vi "TeleopTest.vi"(11 "Call Context":T5) -> ()   [LabVIEW 2015]
doc: "This VI is called for each TeleOp packet received from the DS where the robot is not disabled. It is often used to read from the joysticks and update I/O or to update setpoints for timed control loops. It should complete and return within 20 milliseconds or it may miss DS packets."
uses:
  <vilib>/Rock Robotics/WPI/DriverStation/WPI_DriverStationDerivedRobotMode.ctl
  <vilib>/Rock Robotics/WPI/CAN/TalonSRX/WPI_CANTalonSRX_APIControlMode.ctl
  <vilib>/Rock Robotics/WPI/Utilities/WPI_GetSetVariantRefNum.vi
  Robot Global Data.vi
panel:
  out "error out":errorcluster
  in  "Tab Control":T1(tab)
  out "Maximum":dbl
  out "Minimum":dbl
  out "Maximum?":bool
  out "Minimum?":bool
  in  "Max Length":dbl
  out "Length/Data":dbl
  in  "Angle":dbl(knob) scale=0.0..60.0
  in  "LA PID":cluster{"P":dbl, "I":dbl, "D":dbl}
  in  "Other Settings":T2
  in  "Frequency":dbl
  out "ZN PID":cluster{"P":dbl, "I":dbl, "D":dbl}
  in  "Other Settings":T2
  in  "Wheel PID":cluster{"P":dbl, "I":dbl, "D":dbl}
  in  "Ticks/100ms":dbl
  in  "Frequency":dbl
  out "ZN PID":cluster{"P":dbl, "I":dbl, "D":dbl}
  out "Trigger":bool
  out "Collection Trigger":bool
  out "Lower Button":bool
  out "Vision Prep Button":bool
  out "Motor Position":dbl
  out "Launch Speed":dbl
  in  "Cluster":T3={"LA Distance/Tick(inches)"=0.0, "Framerate"=1000, "Initial Velocity"=0.0, "Max Angle"=60, "Sims/angle"=10}
  in  "Aimbot Transformations":T4={"SpinupDuration(10ms)"=100, "ShotDuration(10ms)"=100, "PowerScale"=1.0, "AngleShift"=0}
  out "Vision Prep Button":bool
  out "Lower Button":bool
  in  "Distance":dbl
  out "Vision Distance":dbl
  out "Launch Speed":dbl
  out "Motor Position":dbl
  out "Trigger":bool
  out "Collection Trigger":bool
  in  "Aimbot Transformations":T4={"SpinupDuration(10ms)"=100, "ShotDuration(10ms)"=100, "PowerScale"=1.0, "AngleShift"=0}
  out "Collection Trigger":bool
  out "Trigger":bool
  out "Lower Button":bool
  out "Vision Prep Button":bool
  out "Launch Speed":dbl
  out "Motor Position":dbl
  out "Vision Distance":dbl
  in  "error in (no error)":errorcluster
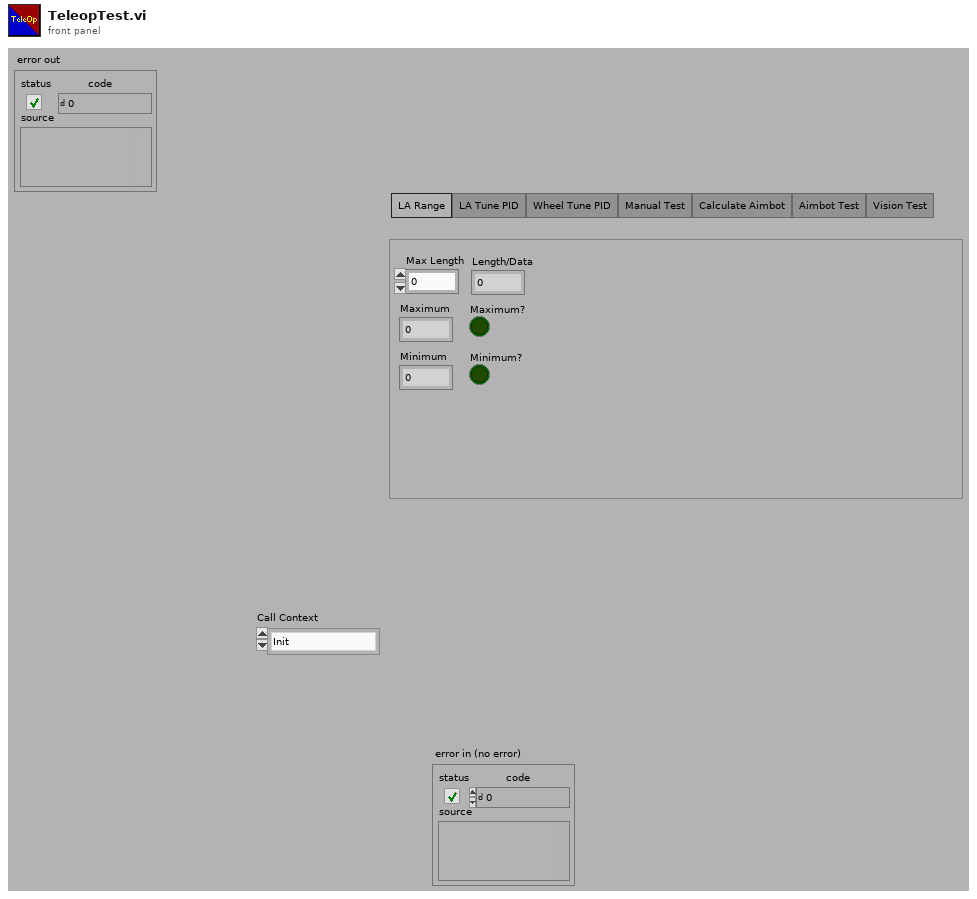
[diagram p1: front panel]
types:
  T1 = enum32{"LA Range", "LA Tune PID", "Wheel Tune PID", "Manual Test", "Calculate Aimbot", "Aimbot Test", "Vision Test"}
  T2 = cluster{"Parameter Slot":u8, "F":dbl, "I Zone":dbl, "Ramp Rate":dbl}
  T3 = cluster{"LA Distance/Tick(inches)":dbl, "Framerate":i32, "Initial Velocity":dbl, "Max Angle":i32, "Sims/angle":i32}
  T4 = cluster{"SpinupDuration(10ms)":i32, "ShotDuration(10ms)":i32, "PowerScale":dbl, "AngleShift":i32}
  T5 = typedef "WPI_DriverStationDerivedRobotMode.ctl" = enum16{"Init", "Execute", "Stop"}
  T6 = typedef "WPI_JoystickDevRef.ctl" = cluster{"Device":T7}
  T7 = typedef "WPI_JoystickDeviceEnum.ctl" = enum16{"USB 0", "USB 1", "USB 2", "USB 3", "USB 4", "USB 5"}
  T8 = typedef "WPI_CANTalonSRX_APIControlMode.ctl" = enum8{"Percent VBus", "Speed", "Position", "Slave", "Unchanged / Invalid", "Voltage Compensation", "Current", "Motion Profile"}
  T9 = cluster{"Joystick":dbl, "LowerButton":bool, "VisionPrepButton":bool, "Aimbot?":bool}
  T10 = cluster{"Framerate":i32, "Initial Velocity":dbl, "Max Angle":i32, "Min Angle":i32, "Sims/angle":i32, "Full Path":path, "Partial Path":path}
  T11 = cluster{"Ball Diameter(in)":dbl, "Air Density(g/in^3)":dbl, "Drag coefficient":dbl, "Ball Mass(g)":dbl, "gravity(in/s^2)":dbl, "Minimum Goal Height(in)":dbl, "Maximum Goal Height(in)":dbl}
  T12 = cluster{"Distance from Pivot Point to Drive Mount(in)":dbl, "Distance from Pivot Point to Arm Mount(in)":dbl, "Distance from Pivot Point to Launcher(in)":dbl, "Distance from Pivot Point to Camera(in)":dbl, "WheelEncoder Ticks/Revolution":dbl, "Wheel Radius":dbl, "Triangle Angle(degrees)":dbl, "Minimum LA Distance(inches)":dbl, "LA Distance/Tick(inches)":dbl}
  T13 = cluster{"Axes[0]":dbl, "Axes[1]":dbl, "Axes[2]":dbl, "Axes[3]":dbl, "Axes[4]":dbl, "Axes[5]":dbl, "Axes[6]":dbl, "Axes[7]":dbl, "Axes[8]":dbl}
  T14 = typedef "WPI_DigitalInputDevRef.ctl" = cluster{"DevStatus":errorcluster, "DIO Channel":T15}
  T15 = typedef "FPGA_DIOChannel.ctl" = enum8{"DIO 0", "DIO 1", "DIO 2", "DIO 3", "DIO 4", "DIO 5", "DIO 6", "DIO 7", "DIO 8", "DIO 9", "DIO MXP 0", "DIO MXP 1", "DIO MXP 2", "DIO MXP 3", "DIO MXP 4", "DIO MXP 5", "DIO MXP 6", "DIO MXP 7", "DIO MXP 8", "DIO MXP 9", "DIO MXP 10", "DIO MXP 11", "DIO MXP 12", "DIO MXP 13", "DIO MXP 14", "DIO MXP 15", "Invalid"}
  T16 = typedef "WPI_MotorControlDeviceRef.ctl" = cluster{"DeviceStatus":errorcluster, "Type":T17, "PWM":cluster{"PWM Channel":T18, "DeadBand":T19}, "CAN":cluster{"Device Number":u8, "Control Mode":T20, "Semaphore":T21, "Max Vout":dbl, "TalonSRX Control Mode":T8}, "Invert":bool}
  T17 = typedef "WPI_MotorControlType.ctl" = enum16{"PWM", "CAN", "CANTalonSRX"}
  T18 = typedef "FPGA_DIOPWMChannel.ctl" = enum8{"PWM 0", "PWM 1", "PWM 2", "PWM 3", "PWM 4", "PWM 5", "PWM 6", "PWM 7", "PWM 8", "PWM 9", "PWM MXP 0", "PWM MXP 1", "PWM MXP 2", "PWM MXP 3", "PWM MXP 4", "PWM MXP 5", "PWM MXP 6", "PWM MXP 7", "PWM MXP 8", "PWM MXP 9", "Invalid"}
  T19 = typedef "WPI_PWMDeadband.ctl" = cluster{"Name":string, "maxPositivePwm":i32, "minPositivePwm":i32, "centerPwm":i32, "maxNegativePwm":i32, "minNegativePwm":i32, "angularRange":u16}
  T20 = typedef "WPI_CANJaguar_ControlMode.ctl" = enum8{"Percent VBus", "Current", "Speed", "Position", "Voltage"}
  T21 = typedef "Semaphore RefNum" = refnum<k1>
  T22 = typedef "WPI_PotentiometerDevRef.ctl" = cluster{"DevStatus":errorcluster, "Analog Channel":T23, "Invert Output":bool}
  T23 = typedef "FPGA_AIChannel.ctl" = enum8{"AI 0", "AI 1", "AI 2", "AI 3", "AI MXP 0", "AI MXP 1", "AI MXP 2", "AI MXP 3", "Invalid"}
  T24 = cluster{"Buttons[0]":bool, "Buttons[1]":bool, "Buttons[2]":bool, "Buttons[3]":bool, "Buttons[4]":bool, "Buttons[5]":bool, "Buttons[6]":bool, "Buttons[7]":bool, "Buttons[8]":bool}
  T25 = cluster{"Angle":dbl, "Distance":dbl, "x":dbl, "y":dbl}
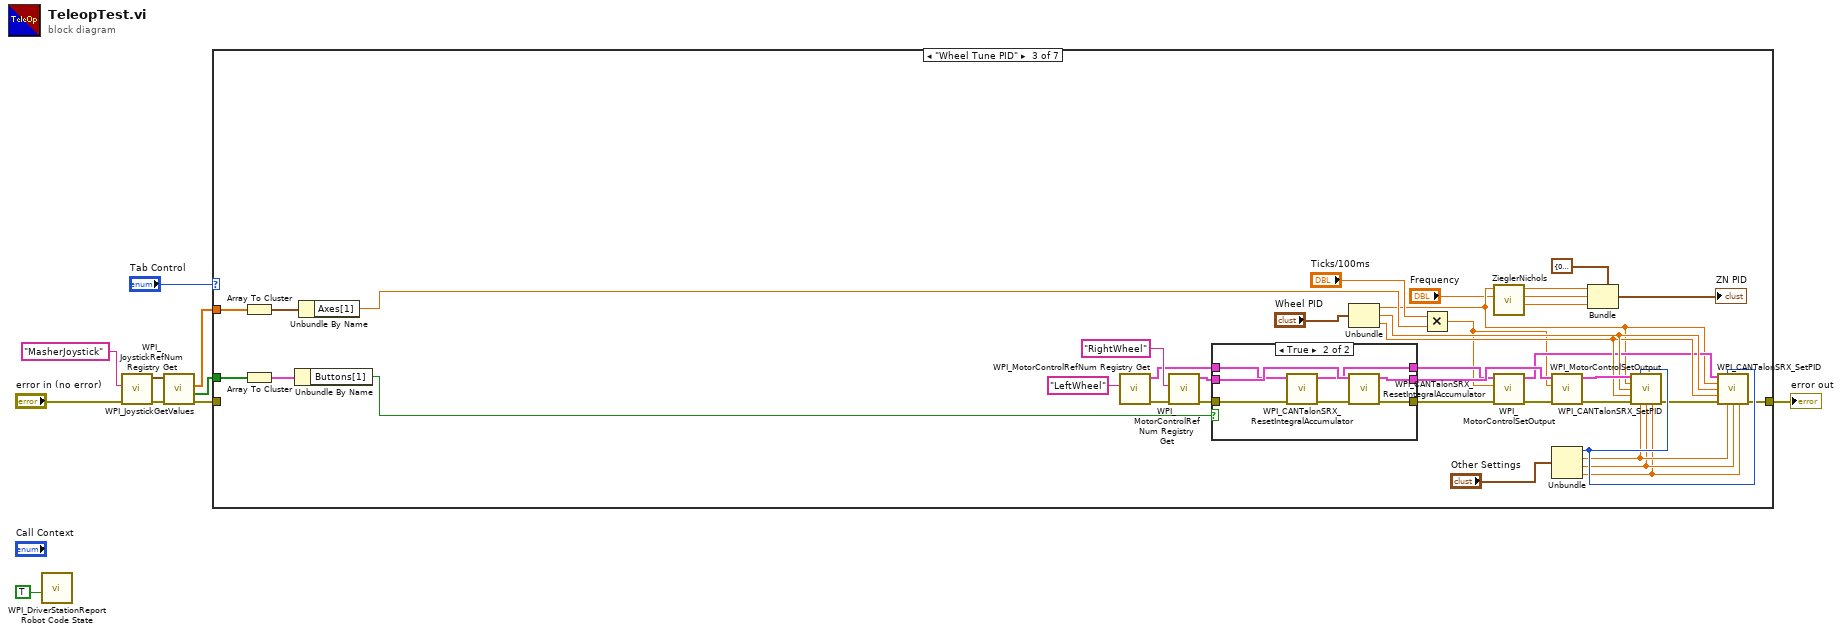
[diagram p0: block diagram]
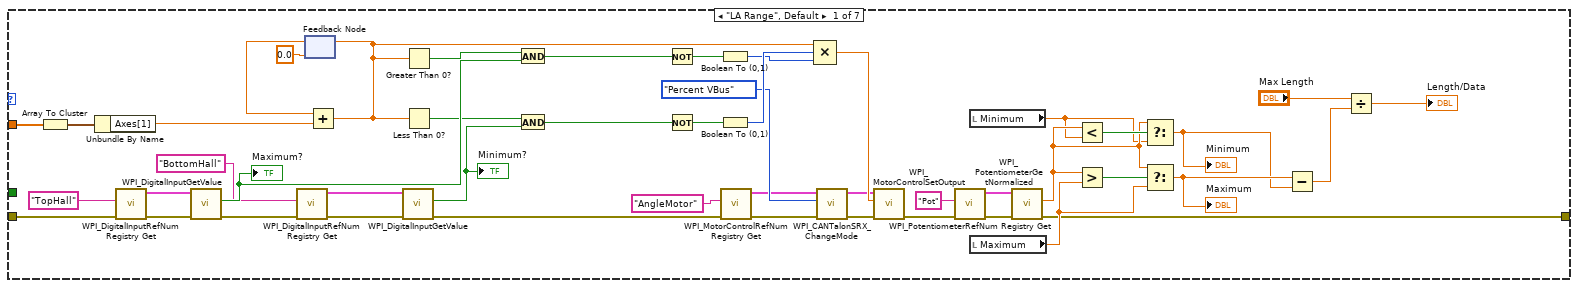
[diagram p2: hidden frame]
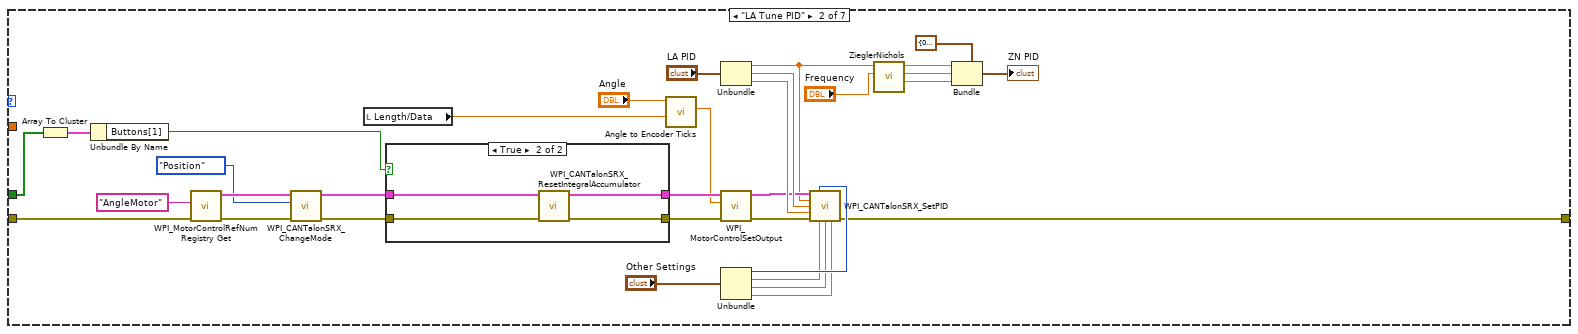
[diagram p3: hidden frame]
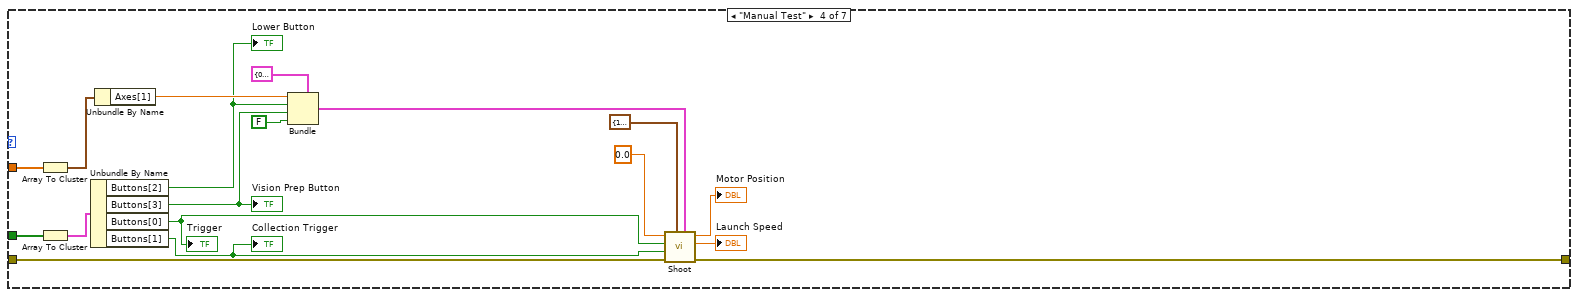
[diagram p6: hidden frame]
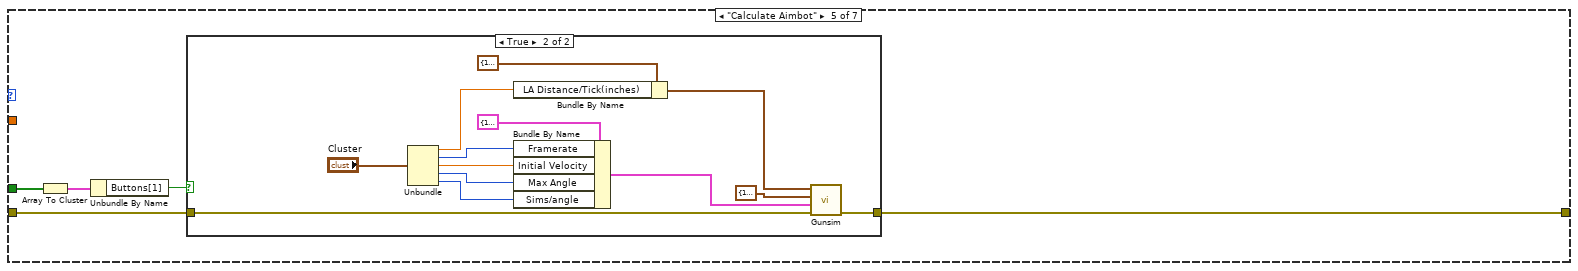
[diagram p7: hidden frame]
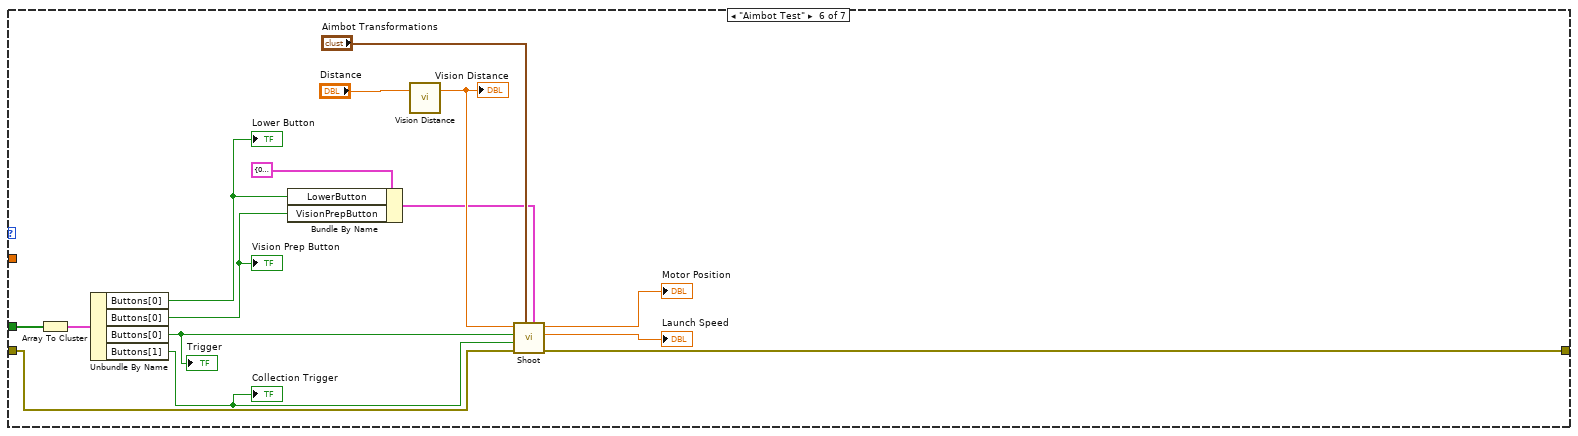
[diagram p9: hidden frame]
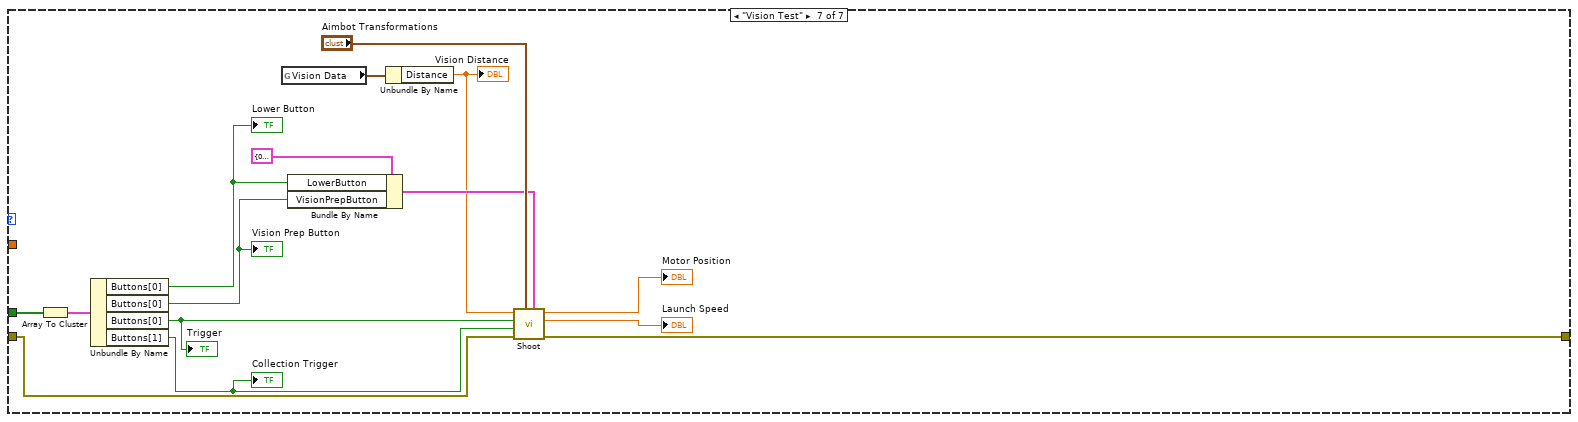
[diagram p10: hidden frame]
diagram:
  n1 = call <vilib>:"WPI_DriverStationReport Robot Code State.vi"("TeleOp"=TRUE ("Autonomous")) -> ()  [unwired: 10 in, 1 out]
  n2 = call <vilib>:"WPI_JoystickRefNum Registry Get.vi"("error in (no error)"="error in (no error)", "refnum name"="MasherJoystick") -> ("error out"=w7:errorcluster, "JoystickDevRef"=w8:T6)  [unwired: 8 in]
  n3 = call <vilib>:"WPI_JoystickGetValues.vi"("error in (no error)"=w7, "JoystickDevRef"=w8) -> ("error out"=w5:errorcluster, "Buttons"=w4:bool[], "Axes"=w3:dbl[])  [unwired: 5 in, 2 out]
  n4 = case shown="\"Wheel Tune PID\"" "Tab Control" {
    tunnel: w5 -> [w24 w86 _ w149 w164 w189 w201]
    tunnel: w4 -> [_ w88 w126 w150 w166 w188 w200]
    tunnel: w3 -> [w49 _ w109 w151 _ _ _]
    tunnel: [w11 w58 w97 w145 w163 w182 w197] -> w1
    frame "LA Range", Default {
      n5 = Array To Cluster(array=w49) -> (cluster=w48:T13)
      n6 = Unbundle By Name(w48) -> ("Axes[1]"=w22:dbl)
      n7 = call <vilib>:"WPI_DigitalInputRefNum Registry Get.vi"("error in (no error)"=w24, "refnum name"="TopHall") -> ("error out"=w31:errorcluster, "DigitalInputDevRef"=w32:T14)  [unwired: 8 in]
      n8 = call <vilib>:"WPI_DigitalInputGetValue.vi"("error in (no error)"=w31, "DigitalInputDevRef"=w32) -> ("error out"=w25:errorcluster, "Value"=w43:bool)  [unwired: 7 in, 1 out]
      "Maximum?" <- w43
      n9 = call <vilib>:"WPI_DigitalInputRefNum Registry Get.vi"("error in (no error)"=w25, "refnum name"="BottomHall") -> ("error out"=w28:errorcluster, "DigitalInputDevRef"=w29:T14)  [unwired: 8 in]
      n10 = feedback #1(0.0) -> (w23:dbl)
      n11 = Add(x=w23, y=w22) -> (x+y=w34:dbl)
      n12 = feedback-in #1(w34) -> ()
      n13 = call <vilib>:"WPI_DigitalInputGetValue.vi"("error in (no error)"=w28, "DigitalInputDevRef"=w29) -> ("error out"=w26:errorcluster, "Value"=w40:bool)  [unwired: 7 in, 1 out]
      "Minimum?" <- w40
      n14 = Greater Than 0?(x=w34) -> (x > 0?=w44:bool)
      n15 = Less Than 0?(x=w34) -> (x < 0?=w39:bool)
      n16 = And(x=w44, y=w43) -> (x .and. y?=w42:bool)
      n17 = And(x=w39, y=w40) -> (x .and. y?=w41:bool)
      n18 = Not(x=w42) -> (.not. x?=w35:bool)
      n19 = Not(x=w41) -> (.not. x?=w38:bool)
      n20 = Boolean To (0,1)(Boolean=w35) -> (0, 1=w36:i16)
      n21 = Boolean To (0,1)(Boolean=w38) -> (0, 1=w37:i16)
      n22 = call <vilib>:"WPI_MotorControlRefNum Registry Get.vi"("error in (no error)"=w26, "refnum name"="AngleMotor") -> ("error out"=w15:errorcluster, "MotorControlDevRef"=w14:T16)  [unwired: 8 in]
      n23 = Compound Arithmetic op=MULTIPLY(w34, w37, w36) -> (w27:dbl)
      n24 = call <vilib>:"WPI_CANTalonSRX_ChangeMode.vi"("error in (no error)"=w15, "Control Mode"=WPI_CANTalonSRX_APIControlMode."Percent VBus", "CAN Talon SRX Ref"=w14) -> ("error out"=w12:errorcluster, "CAN Talon SRX Ref"=w13:T16)  [unwired: 7 in]
      n25 = call <vilib>:"WPI_MotorControlSetOutput.vi"("error in (no error)"=w12, "Output"=w27, "MotorControlDevRef"=w13) -> ("error out"=w45:errorcluster)  [unwired: 6 in, 2 out]
      n26 = call <vilib>:"WPI_PotentiometerRefNum Registry Get.vi"("error in (no error)"=w45, "refnum name"="Pot") -> ("error out"=w56:errorcluster, "PotDevRef"=w57:T22)  [unwired: 8 in]
      n27 = local read "Minimum"() -> (w50:dbl)
      n28 = local read "Maximum"() -> (w51:dbl)
      n29 = call <vilib>:"WPI_PotentiometerGetNormalized.vi"("error in"=w56, "PotDevRef"=w57) -> ("error out"=w11:errorcluster, "Normalized Value"=w52:dbl)  [unwired: 7 in, 1 out]
      n30 = Less?(x=w52, y=w50) -> (x < y?=w53:bool)
      n31 = Greater?(x=w52, y=w51) -> (0:w54:bool)
      n32 = Select(t=w52, s=w53, f=w50) -> (s? t:f=w20:dbl)
      "Minimum" <- w20
      n33 = Select(t=w52, s=w54, f=w51) -> (s? t:f=w21:dbl)
      "Maximum" <- w21
      n34 = Subtract(x=w21, y=w20) -> (x-y=w19:dbl)
      n35 = Divide(x="Max Length", y=w19) -> (x/y=→"Length/Data":dbl)
    }
    frame "LA Tune PID" {
      n36 = Array To Cluster(array=w88) -> (cluster=w89:T24)
      n37 = Unbundle By Name(w89) -> ("Buttons[1]"=w87:bool)
      n38 = call <vilib>:"WPI_MotorControlRefNum Registry Get.vi"("error in (no error)"=w86, "refnum name"="AngleMotor") -> ("error out"=w69:errorcluster, "MotorControlDevRef"=w71:T16)  [unwired: 8 in]
      n39 = call <vilib>:"WPI_CANTalonSRX_ChangeMode.vi"("error in (no error)"=w69, "Control Mode"=WPI_CANTalonSRX_APIControlMode."Position", "CAN Talon SRX Ref"=w71) -> ("error out"=w68:errorcluster, "CAN Talon SRX Ref"=w70:T16)  [unwired: 7 in]
      n40 = local read "Length/Data"() -> (w77:dbl)
      n41 = case shown="True" w87 {
        tunnel: w68 -> [w92 w96]
        tunnel: [w92 w95] -> w85
        tunnel: w70 -> [w91 w94]
        tunnel: [w91 w93] -> w80
        frame False {
        }
        frame True {
          n42 = call <vilib>:"WPI_CANTalonSRX_ResetIntegralAccumulator.vi"("error in (no error)"=w96, "CAN Talon SRX Ref"=w94) -> ("error out"=w95:errorcluster, "CAN Talon SRX Ref"=w93:T16)  [unwired: 8 in]
        }
      }
      n43 = call "Angle to Encoder Ticks.vi"("Length/Rotation"=w77, "Angle(degrees)"="Angle") -> ("Rotations"=w79:dbl)  [unwired: 9 in]
      n44 = Unbundle("LA PID") -> ("P"=w65:dbl, "I"=w84:dbl, "D"=w83:dbl)
      n45 = call <vilib>:"WPI_MotorControlSetOutput.vi"("error in (no error)"=w85, "Output"=w79, "MotorControlDevRef"=w80) -> ("error out"=w82:errorcluster, "MotorControlDevRef"=w81:T16)  [unwired: 6 in, 1 out]
      n46 = Unbundle("Other Settings") -> ("Parameter Slot"=w75:u8, "F"=w74:dbl, "I Zone"=w73:dbl, "Ramp Rate"=w72:dbl)
      n47 = call <vilib>:"WPI_CANTalonSRX_SetPID.vi"("CAN Talon SRX Ref"=w81, "Parameter Slot"=w75, "P"=w65, "I"=w84, "D"=w83, "error in (no error)"=w82, "F"=w74, "I Zone"=w73, "Ramp Rate"=w72) -> ("error out"=w58:errorcluster)  [unwired: 5 in, 1 out]
      n48 = call "ZieglerNichols.vi"("Pc"="Frequency", "Kc"=w65) -> ("Kd"=w60:dbl, "Ki"=w61:dbl, "Kp"=w62:dbl)  [unwired: 3 in]
      n49 = Bundle(cluster=cluster{"P":dbl, "I":dbl, "D":dbl} {"P"=0.0, "I"=0.0, "D"=0.0} ("LA PID"), "P"=w62, "I"=w61, "D"=w60) -> (→"ZN PID":cluster{"P":dbl, "I":dbl, "D":dbl})
    }
    frame "Wheel Tune PID" {
      n50 = Array To Cluster(array=w109) -> (cluster=w110:T13)
      n51 = Array To Cluster(array=w126) -> (cluster=w127:T24)
      n52 = Unbundle By Name(w127) -> ("Buttons[1]"=w125:bool)
      n53 = Unbundle By Name(w110) -> ("Axes[1]"=w108:dbl)
      n54 = call <vilib>:"WPI_MotorControlRefNum Registry Get.vi"("refnum name"="LeftWheel") -> ("error out"=w122:errorcluster, "MotorControlDevRef"=w123:T16)  [unwired: 9 in]
      n55 = call <vilib>:"WPI_MotorControlRefNum Registry Get.vi"("error in (no error)"=w122, "refnum name"="RightWheel") -> ("error out"=w133:errorcluster, "MotorControlDevRef"=w132:T16)  [unwired: 8 in]
      n56 = case shown="True" w125 {
        tunnel: w133 -> [w137 w141]
        tunnel: [w137 w144] -> w113
        tunnel: w132 -> [w136 w143]
        tunnel: [w136 w142] -> w128
        tunnel: w123 -> [w135 w139]
        tunnel: [w135 w138] -> w114
        frame False {
        }
        frame True {
          n57 = call <vilib>:"WPI_CANTalonSRX_ResetIntegralAccumulator.vi"("error in (no error)"=w141, "CAN Talon SRX Ref"=w139) -> ("error out"=w140:errorcluster, "CAN Talon SRX Ref"=w138:T16)  [unwired: 8 in]
          n58 = call <vilib>:"WPI_CANTalonSRX_ResetIntegralAccumulator.vi"("error in (no error)"=w140, "CAN Talon SRX Ref"=w143) -> ("error out"=w144:errorcluster, "CAN Talon SRX Ref"=w142:T16)  [unwired: 8 in]
        }
      }
      n59 = Unbundle("Wheel PID") -> ("P"=w100:dbl, "I"=w121:dbl, "D"=w120:dbl)
      n60 = Multiply(x="Ticks/100ms", y=w108) -> (x*y=w106:dbl)
      n61 = call "ZieglerNichols.vi"("Pc"="Frequency", "Kc"=w100) -> ("Kd"=w104:dbl, "Ki"=w103:dbl, "Kp"=w102:dbl)  [unwired: 3 in]
      n62 = call <vilib>:"WPI_MotorControlSetOutput.vi"("error in (no error)"=w113, "Output"=w106, "MotorControlDevRef"=w114) -> ("error out"=w112:errorcluster, "MotorControlDevRef"=w111:T16)  [unwired: 6 in, 1 out]
      n63 = call <vilib>:"WPI_MotorControlSetOutput.vi"("error in (no error)"=w112, "Output"=w106, "MotorControlDevRef"=w128) -> ("error out"=w130:errorcluster, "MotorControlDevRef"=w129:T16)  [unwired: 6 in, 1 out]
      n64 = Unbundle("Other Settings") -> ("Parameter Slot"=w118:u8, "F"=w117:dbl, "I Zone"=w116:dbl, "Ramp Rate"=w115:dbl)
      n65 = Bundle(cluster=cluster{"P":dbl, "I":dbl, "D":dbl} {"P"=0.0, "I"=0.0, "D"=0.0} ("LA PID"), "P"=w102, "I"=w103, "D"=w104) -> (→"ZN PID":cluster{"P":dbl, "I":dbl, "D":dbl})
      n66 = call <vilib>:"WPI_CANTalonSRX_SetPID.vi"("CAN Talon SRX Ref"=w129, "Parameter Slot"=w118, "P"=w100, "I"=w121, "D"=w120, "error in (no error)"=w130, "F"=w117, "I Zone"=w116, "Ramp Rate"=w115) -> ("error out"=w98:errorcluster)  [unwired: 5 in, 1 out]
      n67 = call <vilib>:"WPI_CANTalonSRX_SetPID.vi"("CAN Talon SRX Ref"=w111, "Parameter Slot"=w118, "P"=w100, "I"=w121, "D"=w120, "error in (no error)"=w98, "F"=w117, "I Zone"=w116, "Ramp Rate"=w115) -> ("error out"=w97:errorcluster)  [unwired: 5 in, 1 out]
    }
    frame "Manual Test" {
      n68 = Array To Cluster(array=w151) -> (cluster=w156:T13)
      n69 = Array To Cluster(array=w150) -> (cluster=w162:T24)
      n70 = Unbundle By Name(w162) -> ("Buttons[2]"=w153:bool, "Buttons[3]"=w152:bool, "Buttons[0]"=w154:bool, "Buttons[1]"=w161:bool)
      "Trigger" <- w154
      "Collection Trigger" <- w161
      "Lower Button" <- w153
      "Vision Prep Button" <- w152
      n71 = Unbundle By Name(w156) -> ("Axes[1]"=w155:dbl)
      n72 = Bundle(cluster=T9 {"Joystick"=0.0, "LowerButton"=FALSE, "VisionPrepButton"=FALSE, "Aimbot?"=TRUE} ("Manual Control"), "Joystick"=w155, "LowerButton"=w153, "VisionPrepButton"=w152, "Aimbot?"=FALSE) -> (w157:T9)
      n73 = call "Shoot.vi"("Manual Control"=w157, "Aimbot Transformations"=T4 {"SpinupDuration(10ms)"=100, "ShotDuration(10ms)"=100, "PowerScale"=1.0, "AngleShift"=0} ("Override Data"), "error in"=w149, "Collection Trigger"=w161, "Trigger"=w154, "Vision Distance"=0.0) -> ("error out"=w145:errorcluster, "LaunchSpeed(t/100ms)"=→"Launch Speed":dbl, "AngleMotorPosition(t)"=→"Motor Position":dbl)  [unwired: 3 in]
    }
    frame "Calculate Aimbot" {
      n74 = Array To Cluster(array=w166) -> (cluster=w167:T24)
      n75 = Unbundle By Name(w167) -> ("Buttons[1]"=w165:bool)
      n76 = case shown="True" w165 {
        tunnel: w164 -> [w168 w170]
        tunnel: [w168 w169] -> w163
        frame False {
        }
        frame True {
          n77 = Unbundle("Cluster") -> ("LA Distance/Tick(inches)"=w174:dbl, "Framerate"=w175:i32, "Initial Velocity"=w178:dbl, "Max Angle"=w177:i32, "Sims/angle"=w176:i32)
          n78 = Bundle By Name(cluster=T12 {"Distance from Pivot Point to Drive Mount(in)"=16.25, "Distance from Pivot Point to Arm Mount(in)"=5.625, "Distance from Pivot Point to Launcher(in)"=31.125, "Distance from Pivot Point to Camera(in)"=25.625, "WheelEncoder Ticks/Revolution"=0.00048828125, "Wheel Radius"=4.0, "Triangle Angle(degrees)"=51.75, "Minimum LA Distance(inches)"=12.125, "LA Distance/Tick(inches)"=0.0} ("Robot Constants"), "LA Distance/Tick(inches)"=w174) -> (w172:T12)
          n79 = Bundle By Name(cluster=T10 {"Framerate"=1000, "Initial Velocity"=0.0, "Max Angle"=60, "Min Angle"=0, "Sims/angle"=10, "Full Path"=path "/home/lvuser/allranges", "Partial Path"=path "/home/lvuser/ranges"} ("Parameters"), "Framerate"=w175, "Initial Velocity"=w178, "Max Angle"=w177, "Sims/angle"=w176) -> (w171:T10)
          n80 = call "Gunsim.vi"("error in (no error)"=w170, "Parameters"=w171, "Other Constants"=T11 {"Ball Diameter(in)"=10.0, "Air Density(g/in^3)"=0.02, "Drag coefficient"=0.5, "Ball Mass(g)"=300.0, "gravity(in/s^2)"=-386.09, "Minimum Goal Height(in)"=90.0, "Maximum Goal Height(in)"=104.0}, "Robot Constants"=w172) -> ("error out"=w169:errorcluster)  [unwired: 7 in]
        }
      }
    }
    frame "Aimbot Test" {
      n81 = Array To Cluster(array=w188) -> (cluster=w192:T24)
      n82 = Unbundle By Name(w192) -> ("Buttons[0]"=w184:bool, "Buttons[0]"=w185:bool, "Buttons[0]"=w196:bool, "Buttons[1]"=w193:bool)
      "Vision Prep Button" <- w185
      "Lower Button" <- w184
      "Trigger" <- w196
      "Collection Trigger" <- w193
      n83 = Bundle By Name(cluster=T9 {"Joystick"=0.0, "LowerButton"=FALSE, "VisionPrepButton"=FALSE, "Aimbot?"=TRUE} ("Manual Control"), "LowerButton"=w184, "VisionPrepButton"=w185) -> (w183:T9)
      n84 = call "Vision Distance.vi"("Horizontal Distance"="Distance") -> ("Vision Distance"=w190:dbl)  [unwired: 2 in]
      "Vision Distance" <- w190
      n85 = call "Shoot.vi"("Manual Control"=w183, "Aimbot Transformations"="Aimbot Transformations", "error in"=w189, "Collection Trigger"=w193, "Trigger"=w196, "Vision Distance"=w190) -> ("error out"=w182:errorcluster, "LaunchSpeed(t/100ms)"=→"Launch Speed":dbl, "AngleMotorPosition(t)"=→"Motor Position":dbl)  [unwired: 3 in]
    }
    frame "Vision Test" {
      n86 = Array To Cluster(array=w200) -> (cluster=w207:T24)
      n87 = Unbundle By Name(w207) -> ("Buttons[0]"=w203:bool, "Buttons[0]"=w204:bool, "Buttons[0]"=w211:bool, "Buttons[1]"=w208:bool)
      "Vision Prep Button" <- w204
      "Lower Button" <- w203
      "Trigger" <- w211
      "Collection Trigger" <- w208
      n88 = global read "Robot Global Data.vi" "Vision Data"() -> (w199:T25)
      n89 = Bundle By Name(cluster=T9 {"Joystick"=0.0, "LowerButton"=FALSE, "VisionPrepButton"=FALSE, "Aimbot?"=TRUE} ("Manual Control"), "LowerButton"=w203, "VisionPrepButton"=w204) -> (w202:T9)
      n90 = Unbundle By Name(w199) -> ("Distance"=w198:dbl)
      "Vision Distance" <- w198
      n91 = call "Shoot.vi"("Manual Control"=w202, "Aimbot Transformations"="Aimbot Transformations", "error in"=w201, "Collection Trigger"=w208, "Trigger"=w211, "Vision Distance"=w198) -> ("error out"=w197:errorcluster, "LaunchSpeed(t/100ms)"=→"Launch Speed":dbl, "AngleMotorPosition(t)"=→"Motor Position":dbl)  [unwired: 3 in]
    }
  }
  "error out" <- w1
